vi "to string.vi"(8 "error in":errorcluster, 11 "UI Reference configuration in":refnum<class "UI Reference configuration.lvclass">) -> (0 "error out":errorcluster, 1 "data":string, 2 "version":string, 3 "UI Reference configuration out":refnum<class "UI Reference configuration.lvclass">)   [LabVIEW 2013, in "UI Reference configuration.lvclass"]
doc: "Provides an interface for saving a module configuration to a file or other serialized data source. It is recommended that all children of this class store data in two sets--data required for its own initialization, and any data required for parent initialization--and that each implementation uses the <b>Call Parent Method</b> primitive to serialize parent information."
uses:
  UI Reference configuration.lvclass
  <vilib>/NI/Tag Bus Module Framework/module configuration/TBM module configuration.lvclass
  UI Reference configuration.lvclass/UI Reference configuration.ctl
  <vilib>/NI/Tag Bus Module Framework/root configuration/TBM configuration.lvclass
  <vilib>/NI/Tag Bus Module Framework/channel/TBM channel.lvclass
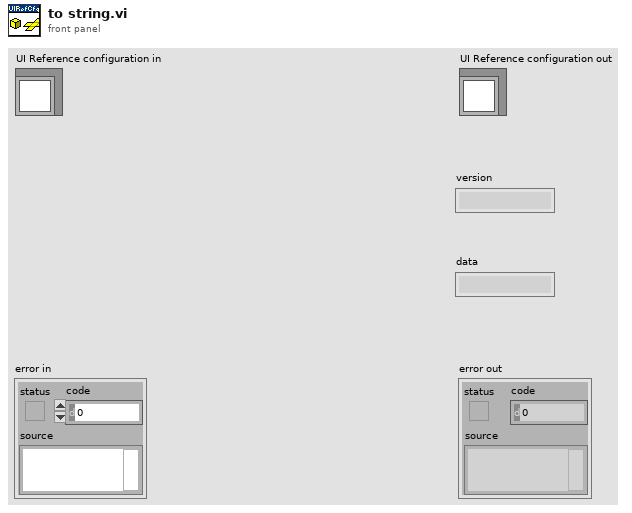
[diagram p1: front panel]
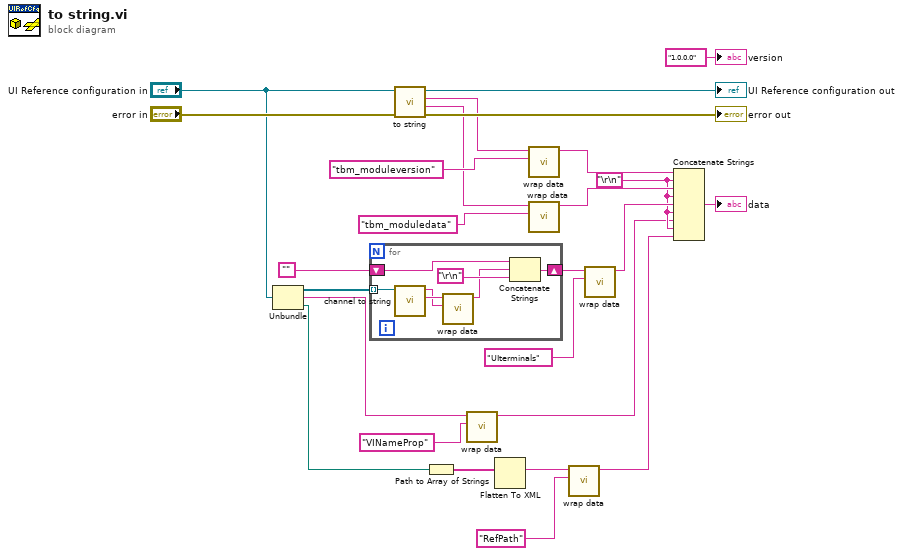
[diagram p0: block diagram]
diagram:
  w6 = "\r\n"
  n1 = Unbundle("UI Reference configuration in") -> (w13:refnum<class "TBM channel.lvclass">[], w2:string, w1:path)
  n2 = for {
    tunnel: w13 -> [w33] mode=indexing
    shift-right: [w29] -> w11
    shift-left: "" -> [w28]
    n3 = call <vilib>:"channel to string.vi"("channel in"=w33) -> ("channel data"=w32:string, "identifier"=w31:string)  [unwired: 9 in]
    n4 = call <vilib>:"wrap data.vi"("identifier"=w31, "data to wrap"=w32) -> ("wrapped data"=w27:string)  [unwired: 9 in]
    n5 = Concatenate Strings(w28, w27, "\r\n") -> (w29:string)
  }
  n6 = call-parent "to string.vi"("error in"="error in", "module configuration in"="UI Reference configuration in") -> ("error out"=→"error out":errorcluster, "data"=w18:string, "version"=w19:string, "module configuration out"=→"UI Reference configuration out":refnum<class "UI Reference configuration.lvclass">)  [unwired: 6 in]
  n7 = Path to Array of Strings(0:w1) -> (2:w5:string[])  [unwired: 1 out]
  n8 = call <vilib>:"wrap data.vi"("identifier"="VINameProp" ("additional identifier"), "data to wrap"=w2) -> ("wrapped data"=w3:string)  [unwired: 9 in]
  n9 = Flatten To XML(anything=w5) -> (xml string=w4:string)
  n10 = call <vilib>:"wrap data.vi"("identifier"="tbm_moduleversion" ("additional identifier"), "data to wrap"=w19) -> ("wrapped data"=w21:string)  [unwired: 9 in]
  n11 = call <vilib>:"wrap data.vi"("identifier"="tbm_moduledata" ("additional identifier"), "data to wrap"=w18) -> ("wrapped data"=w20:string)  [unwired: 9 in]
  n12 = call <vilib>:"wrap data.vi"("identifier"="RefPath" ("additional identifier"), "data to wrap"=w4) -> ("wrapped data"=w8:string)  [unwired: 9 in]
  n13 = call <vilib>:"wrap data.vi"("identifier"="UIterminals" ("additional identifier"), "data to wrap"=w11) -> ("wrapped data"=w15:string)  [unwired: 9 in]
  n14 = Concatenate Strings(w21, w6, w20, w6, w15, w6, w3, w6, w8) -> (→"data":string)
  "version" <- "1.0.0.0" ("version")
